vi "Display.vi"(8 "error in (no error)":errorcluster, 11 "DisplayTetrodes in":refnum<class "DisplayTetrodes.lvclass">) -> (0 "error out":errorcluster, 3 "DisplayTetrodes out":refnum<class "DisplayTetrodes.lvclass">)   [LabVIEW 2011, in "DisplayTetrodes.lvclass"]
uses:
  DisplayTetrodes.lvclass
  <vilib>/Analysis/3filter.llb/Filter Passband Type.ctl
  <vilib>/Analysis/2dsp.llb/Decimate (continuous, DBL).vi
  <vilib>/Analysis/3filter.llb/Butterworth Filter (DBL).vi
  Program Files/National Instruments/LabVIEW 2011/resource/objmgr/ni.dex.rc
  <vilib>/Analysis/NI_AALBase.lvlib
  <vilib>/Analysis/NI_AALPro.lvlib
panel:
  out "STOP ALL":bool
  in  "Tab Control":enum32{"Connection", "Filter", "Display"}(tab)
  in  "Network Stream Writer IP":string(combo)
  out "Connected":bool
  out "% Elems Left":dbl(slide) scale=0.0..100.0
  in  "High Cutoff (Hz)":dbl=6000.0 format="%0.2f"
  in  "Low Cutoff (Hz)":dbl=600.0 format="%0.4f"
  in  "Filter Type":T1=enum."Bandpass"
  in  "FilterData":bool=TRUE
  in  "Decimation Factor":i32=4
  in  "Spacing (microVolts)":dbl=100.0
  in  "DiodeScale":dbl=0.05
  out "Waveform Chart":waveform(dbl)[](graph)
  in  "STOP":bool
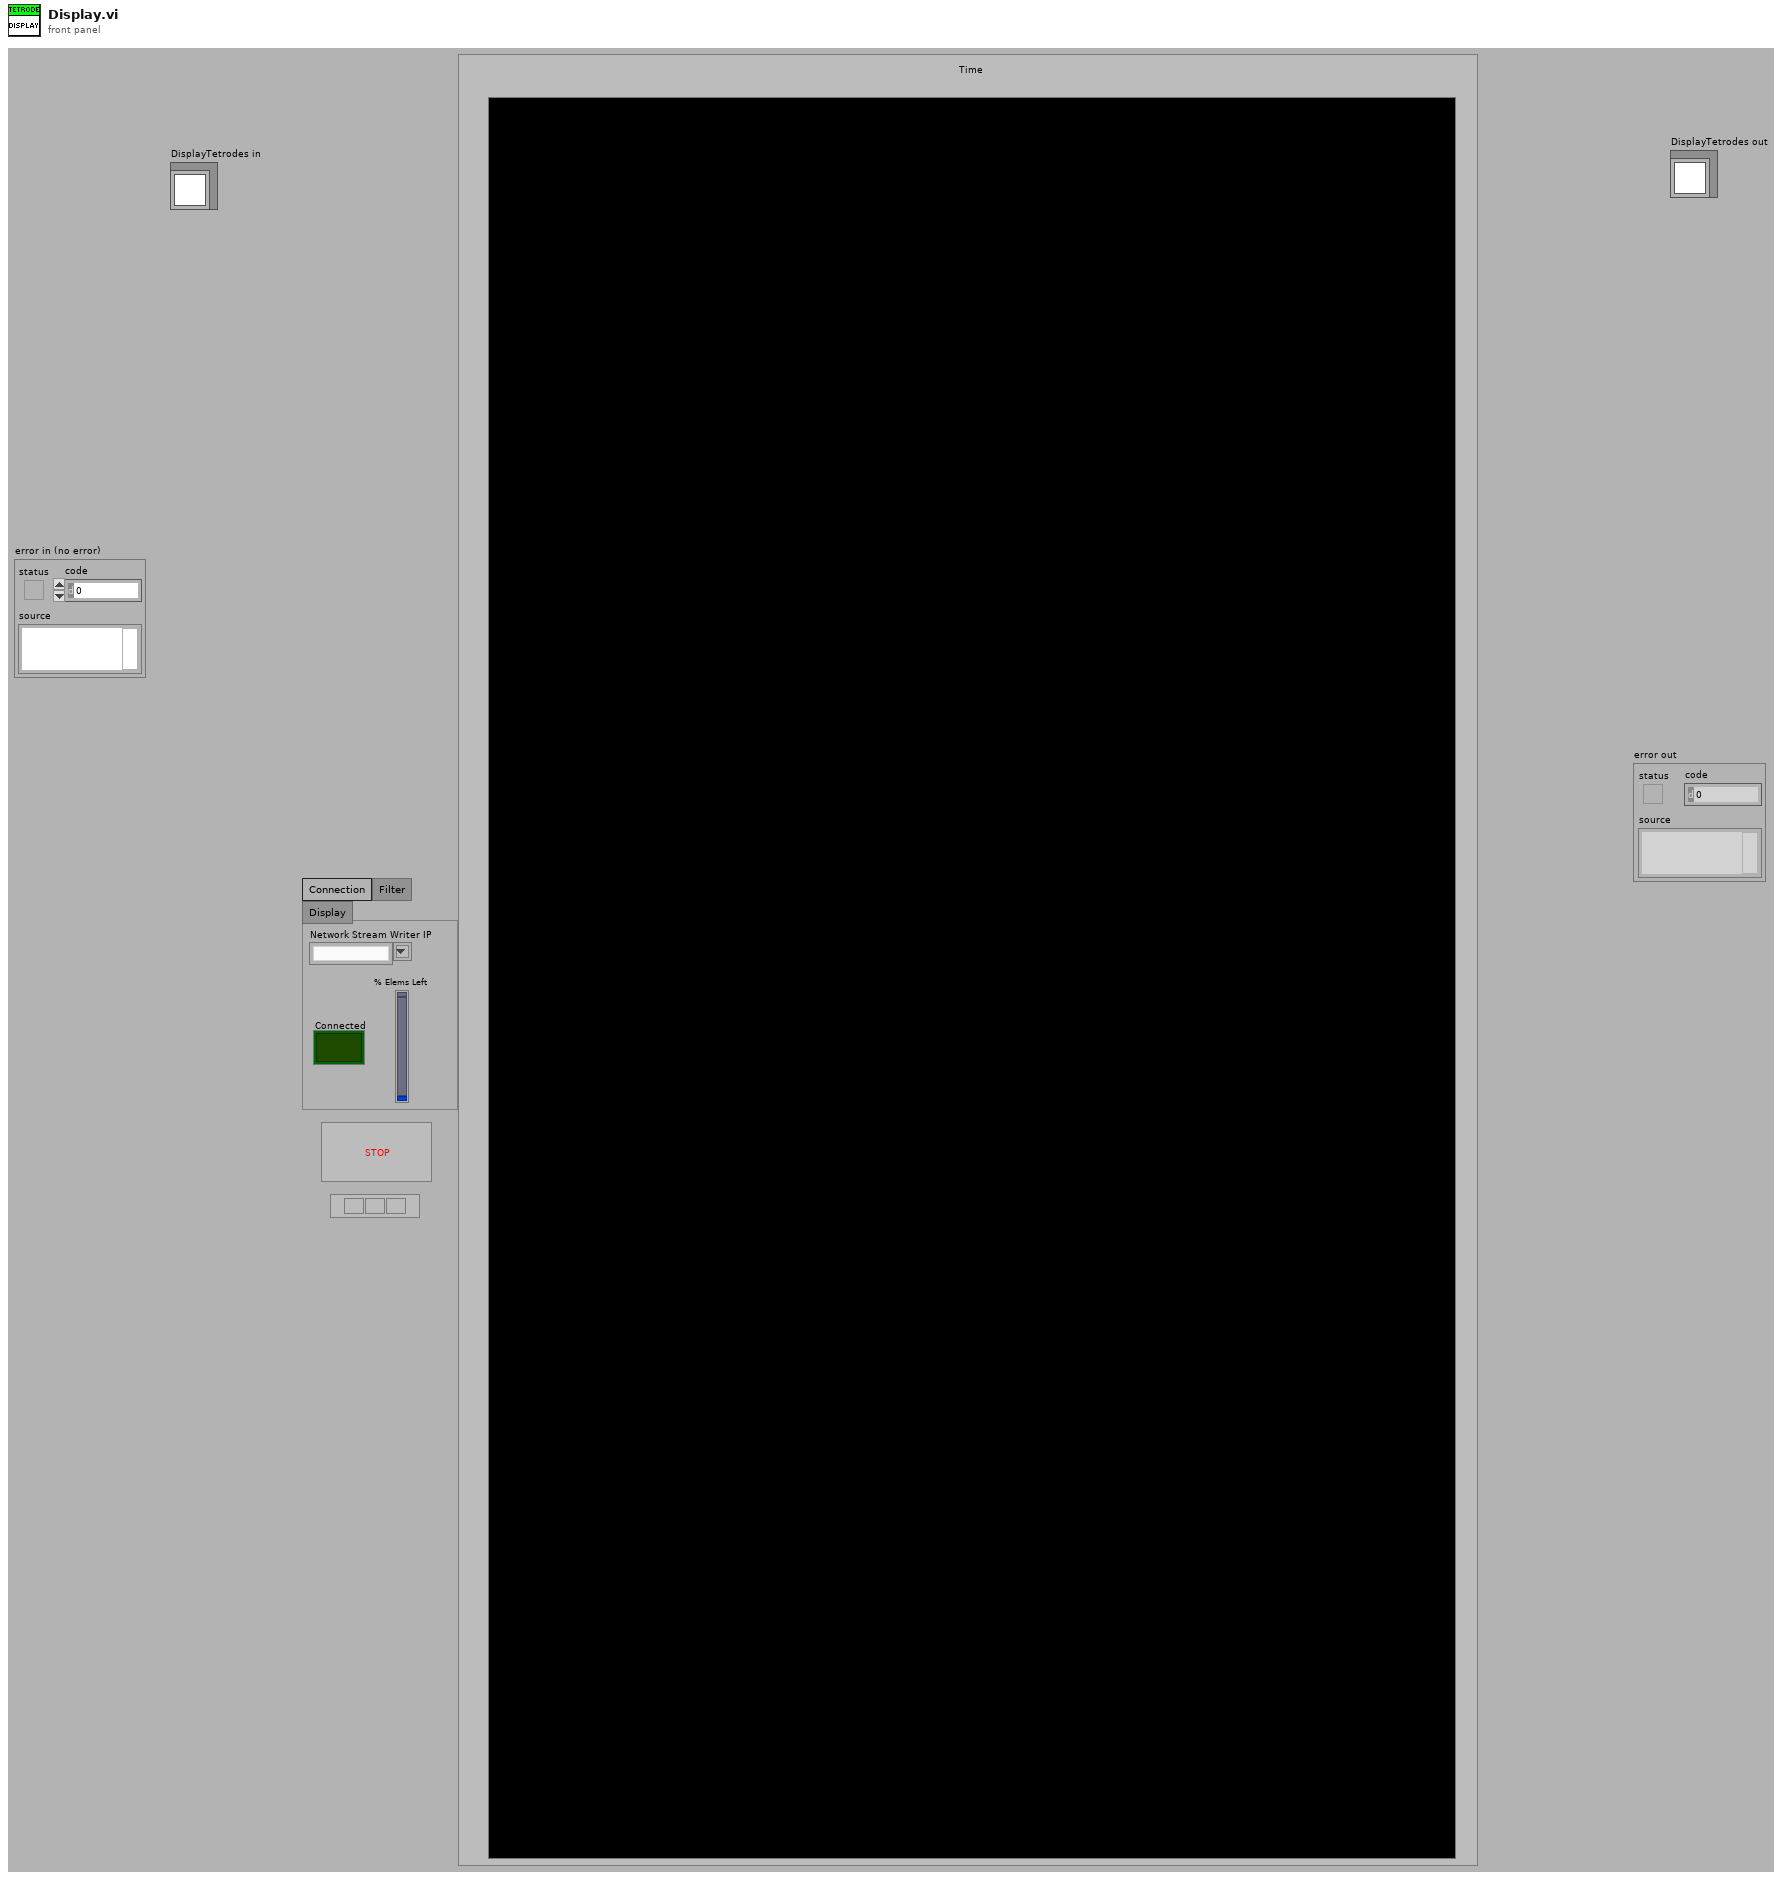
[diagram p1: front panel]
types:
  T1 = typedef "NI_AALBase.lvlib/Filter Passband Type.ctl" = enum32{"Lowpass", "Highpass", "Bandpass", "Bandstop"}
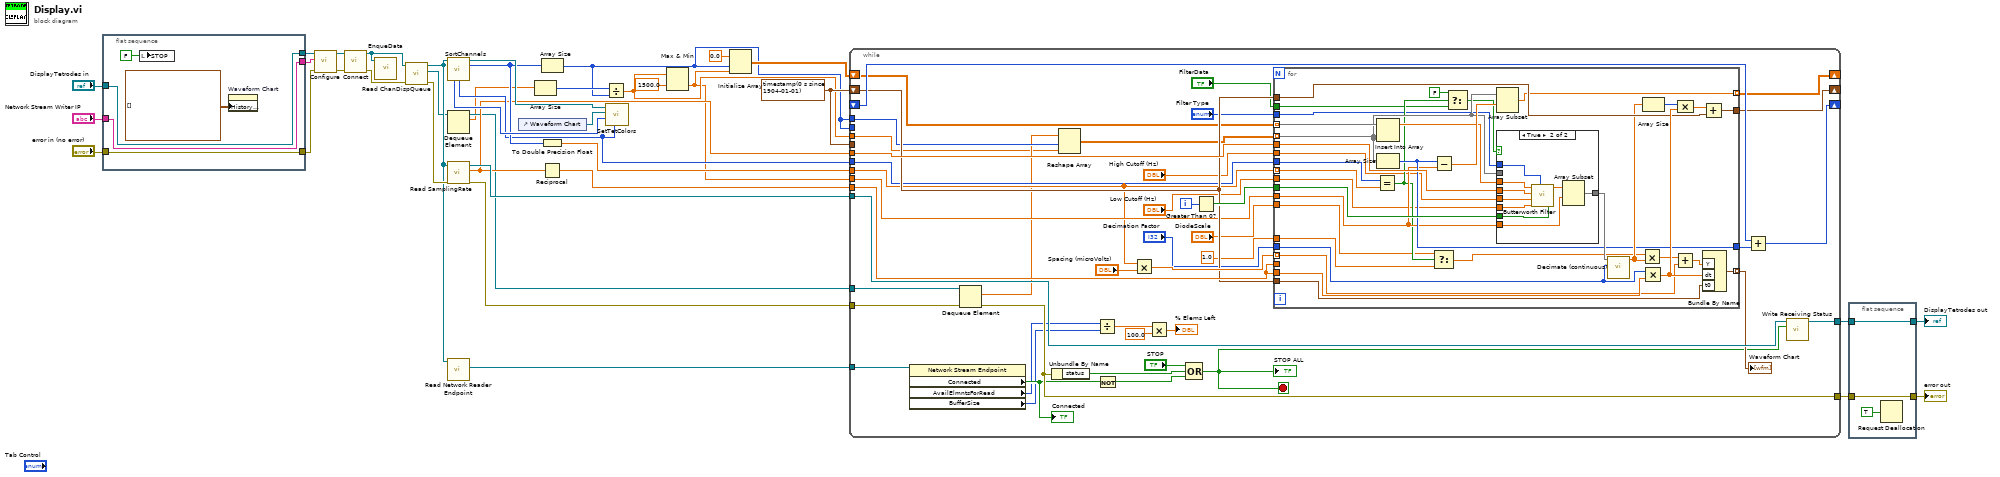
[diagram p0: block diagram]
diagram:
  w22 = timestamp(0 s since 1904-01-01)
  n1 = flat-sequence {
    tunnel: "DisplayTetrodes in" -> [w42]
    tunnel: [w42] -> w29
    tunnel: "Network Stream Writer IP" -> [w41]
    tunnel: [w41] -> w27
    tunnel: "error in (no error)" -> [w40]
    tunnel: [w40] -> w25
    frame #0 {
      n2 = local write "STOP"(FALSE ("STOP")) -> ()
      n3 = property on="Waveform Chart" class="WFChart (strict)"("History Data"=waveform(dbl)[][] []) -> ()  [unwired: 2 in, 2 out]
    }
  }
  n4 = call-dynamic "Configure.vi"("error in (no error)"=w25, "Network Stream Writer IP"=w27, "DataReceiver in"=w29) -> ("error out"=w12:errorcluster, "DataReceiver out"=w13:refnum<class "DisplayTetrodes.lvclass">)  [unwired: 7 in]
  n5 = call-dynamic "Connect.vi"("error in (no error)"=w12, "DataReceiver in"=w13) -> ("error out"=w36:errorcluster, "DataReceiver out"=w37:refnum<class "DisplayTetrodes.lvclass">)  [unwired: 8 in]
  n6 = call-dynamic "EnqueData.vi"("DataReceiver in"=w37) -> ()  [unwired: 9 in, 2 out]
  n7 = call-dynamic "Read ChanDispQueue.vi"("error in (no error)"=w36, "DataReceiver in"=w37) -> ("error out"=w38:errorcluster, "ChanDispQueue"=w8:refnum<queue>, "DataReceiver out"=w15:refnum<class "DisplayTetrodes.lvclass">)  [unwired: 7 in]
  n8 = call-dynamic "SortChannels.vi"("DisplayTetrodes in"=w15) -> ("DisplayTetrodes out"=w20:refnum<class "DisplayTetrodes.lvclass">, "reorderedChanNums"=w18:i32[], "unsortedTetNums"=w19:i32[], "reorderedDiodeChan"=w17:i32)  [unwired: 7 in, 4 out]
  n9 = Dequeue Element(queue=w8) -> (queue out=w7:refnum<queue>, element=w5:dbl[])  [unwired: 2 in, 2 out]
  n10 = call-dynamic "Read SamplingRate.vi"("error in (no error)"=w38, "DataReceiver in"=w15) -> ("error out"=w9:errorcluster, "SamplingRate"=w10:dbl, "DataReceiver out"=w14:refnum<class "DisplayTetrodes.lvclass">)  [unwired: 7 in]
  n11 = call-dynamic "Read Network Reader Endpoint.vi"("DataReceiver in"=w15) -> ("Network Stream Reader Endpoint"=w16:refnum<k21>)  [unwired: 8 in, 2 out]
  n12 = control-ref of="Waveform Chart"() -> (w11:refnum<vi>)
  n13 = Array Size(array=w5) -> (size(s)=w6:i32)
  n14 = Reciprocal(x=w10) -> (1/x=w33:dbl)
  n15 = Array Size(array=w18) -> (size(s)=w4:i32)
  n16 = To Double Precision Float(number=w18) -> (double precision float=w21:dbl[])
  n17 = Divide(x=w6, y=w4) -> (x/y=w3:dbl)
  n18 = call-dynamic "SetTetColors.vi"("Photodiode"=w17, "Unsorted Tet Nums"=w19, "WFChart Refnum"=w11, "DisplayTetrodes in"=w20) -> ()  [unwired: 6 in, 2 out]
  n19 = Max & Min(x=w3, y=1500.0) -> (min(x,y)=w1:dbl)  [unwired: 1 out]
  n20 = Initialize Array(0.0 ("element"), w4, w1) -> (w23:dbl[][])
  n21 = while {
    tunnel: w10 -> [w85]
    tunnel: [w78] -> w35
    tunnel: w9 -> [w82]
    tunnel: w14 -> [w77]
    tunnel: [w79] -> w32
    tunnel: w21 -> [w63]
    tunnel: w33 -> [w72]
    shift-right: [w74] -> _
    shift-left: _ -> [w73]
    tunnel: w22 -> [_]
    shift-right: [w69] -> _
    shift-left: w22 -> [w70]
    shift-right: [w68] -> _
    shift-left: w23 -> [w67]
    tunnel: w1 -> [w66]
    tunnel: w17 -> [w64]
    tunnel: w4 -> [w61]
    tunnel: w4 -> [_]
    tunnel: w16 -> [w58]
    tunnel: w7 -> [w45]
    tunnel: w3 -> [w44]
    i -> [w87]
    stop <- w62 stop-if-true
    n22 = property class="Network Stream Endpoint"(reference=w58) -> ("Connected"=w57:bool, "AvailElmntsForRead"=w50:i32, "BufferSize"=w49:i32)  [unwired: 1 in, 2 out]
    "Connected" <- w57
    n23 = Dequeue Element(queue=w45, error in (no error)=w82) -> (element=w60:dbl[], error out=w78:errorcluster)  [unwired: 1 in, 2 out]
    n24 = Unbundle By Name(w78) -> ("status"=w80:bool)
    n25 = Reshape Array(w60, w61, w44) -> (w59:dbl[][])
    n26 = Divide(x=w50, y=w49) -> (x/y=w48:dbl)
    n27 = Not(x=w57) -> (.not. x?=w76:bool)
    n28 = Multiply(x=w63, y="Spacing (microVolts)") -> (x*y=w83:dbl[])
    n29 = Multiply(x=w48, y=100.0) -> (x*y=→"% Elems Left":dbl)
    n30 = Compound Arithmetic op=OR("STOP", w80, w76) -> (w62:bool)
    "STOP ALL" <- w62
    n31 = Greater Than 0?(x=w87) -> (x > 0?=w86:bool)
    n32 = for {
      tunnel: w59 -> [w102] mode=indexing
      tunnel: w86 -> [w121]
      tunnel: w85 -> [w122]
      tunnel: w83 -> [w109] mode=indexing
      tunnel: w72 -> [_]
      tunnel: [w107] -> w75
      tunnel: w72 -> [w119]
      tunnel: w70 -> [w115]
      tunnel: [w114] -> w71 mode=indexing
      tunnel: w70 -> [w113]
      tunnel: [w112] -> w69
      tunnel: [w105] -> w68 mode=indexing
      tunnel: w67 -> [w104] mode=indexing
      tunnel: w66 -> [w101]
      tunnel: "FilterData" -> [w96]
      tunnel: w64 -> [w99]
      tunnel: w63 -> [w98] mode=indexing
      tunnel: 1.0 ("Scale") -> [w93]
      tunnel: "Filter Type" -> [w92]
      tunnel: "High Cutoff (Hz)" -> [w91]
      tunnel: "Low Cutoff (Hz)" -> [w90]
      tunnel: "Decimation Factor" -> [w89]
      tunnel: "DiodeScale" -> [w88]
      n33 = Equal?(x=w99, y=w98) -> (x = y?=w97:bool)
      n34 = Insert Into Array(array=w104, new element=w102) -> (w103:dbl[])  [unwired: 1 in]
      n35 = Array Size(array=w102) -> (size(s)=w107:i32)
      n36 = Subtract(x=w107, y=w101) -> (x-y=w106:dbl)
      n37 = Select(t=w88, s=w97, f=w93) -> (s? t:f=w100:dbl)
      n38 = Select(t=FALSE, s=w97, f=w96) -> (s? t:f=w94:bool)
      n39 = Array Subset(array=w102, index=w106) -> (w105:dbl[])  [unwired: 1 in]
      n40 = case shown="True" w94 {
        tunnel: w91 -> [_ w132]
        tunnel: w90 -> [_ w131]
        tunnel: w122 -> [_ w130]
        tunnel: w121 -> [_ w129]
        tunnel: w92 -> [_ w128]
        tunnel: [w123 w124] -> w120
        tunnel: w103 -> [_ w127]
        tunnel: w102 -> [w123 _]
        tunnel: w101 -> [_ w125]
        frame False {
        }
        frame True {
          n41 = call-poly <vilib>:"Butterworth Filter.vi"("init/cont (init:F)"=w129, "filter type"=w128, "low cutoff freq: fl"=w131, "high cutoff freq: fh"=w132, "sampling freq: fs"=w130, "X"=w127) -> ("Filtered X"=w126:dbl[])  [unwired: 2 in, 1 out]
          n42 = Array Subset(array=w126, index=w125) -> (w124:dbl[])  [unwired: 1 in]
        }
      }
      n43 = call-poly <vilib>:"Decimate (continuous).vi"("decimating factor"=w89, "X"=w120) -> ("Decimated Array"=w110:dbl[])  [unwired: 8 in, 1 out]
      n44 = Multiply(x=w100, y=w110) -> (x*y=w111:dbl[])
      n45 = Multiply(x=w89, y=w119) -> (x*y=w117:dbl)
      n46 = Array Size(array=w110) -> (size(s)=w118:i32)
      n47 = Add(x=w111, y=w109) -> (x+y=w108:dbl[])
      n48 = Compound Arithmetic op=MULTIPLY(w118, w117) -> (w116:dbl)
      n49 = Add(x=w116, y=w115) -> (x+y=w112:timestamp)
      n50 = Bundle By Name("Y"=w108, "dt"=w117, "t0"=w113) -> (w114:waveform(dbl))  [unwired: 1 in]
    }
    "Waveform Chart" <- w71
    n51 = Add(x=w73, y=w75) -> (x+y=w74:i32)
    n52 = call-dynamic "Write Receiving Status.vi"("Stop Reading"=w62, "DataReceiver in"=w77) -> ("DataReceiver out"=w79:refnum<class "DisplayTetrodes.lvclass">)  [unwired: 8 in, 1 out]
  }
  n53 = flat-sequence {
    tunnel: w35 -> [w135]
    tunnel: [w135] -> w34
    tunnel: w32 -> [w134]
    tunnel: [w134] -> w31
    frame #0 {
      n54 = Request Deallocation(TRUE ("flag")) -> ()
    }
  }
  "error out" <- w34
  "DisplayTetrodes out" <- w31
